vi "forecastUI.vi"(11 "ForecastDisplay in":refnum<class "ForecastDisplay.lvclass">) -> ()   [LabVIEW 2018, in "ForecastDisplay.lvclass"]
uses:
  ForecastDisplay.lvclass
panel:
  out "Waveform Chart":T1(graph)
  out "error out":errorcluster
  in  "error in (no error)":errorcluster
  # "Forecast Display"
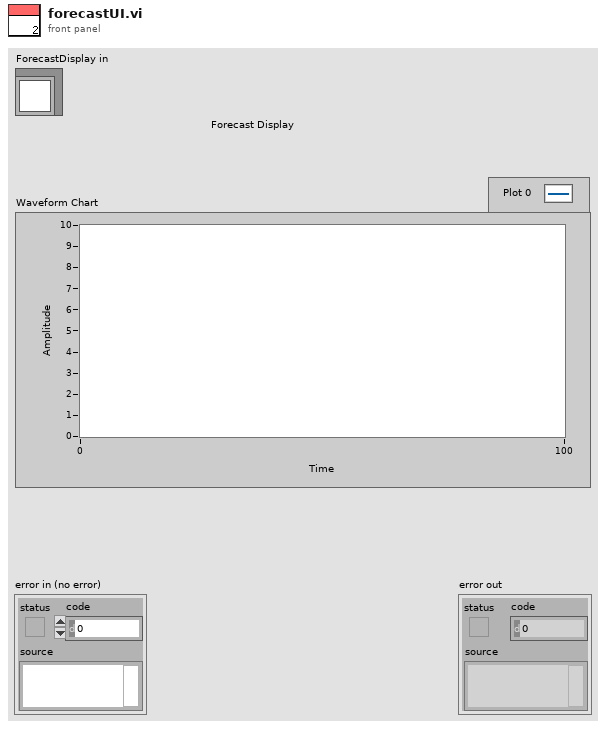
[diagram p1: front panel]
types:
  T1 = cluster{"Temperature":dbl, "Humidity":dbl, "Pressure":dbl}
  T2 = enum16{"Always On", "Always Off", "Off While Running"}
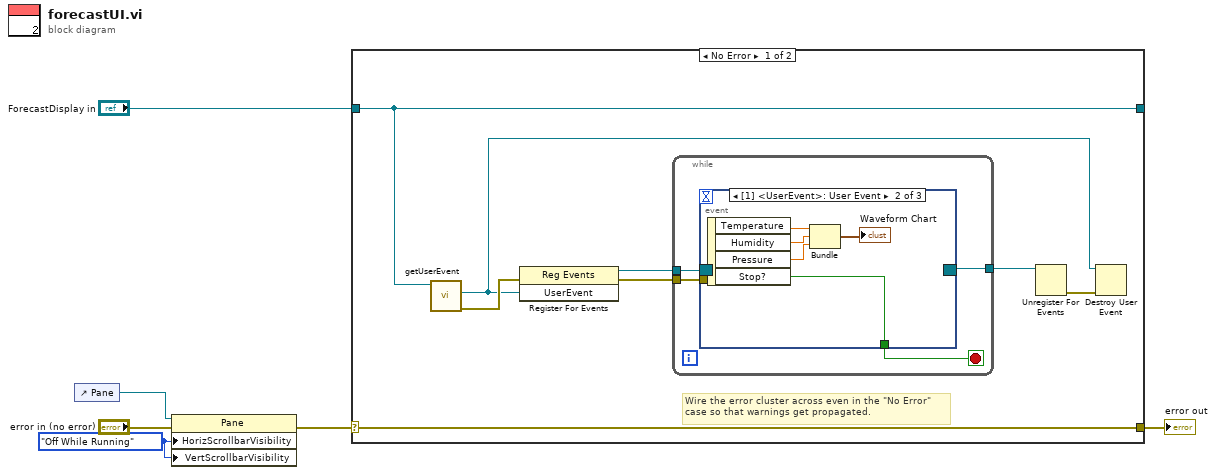
[diagram p0: block diagram]
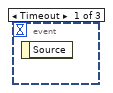
[diagram p2: hidden frame]
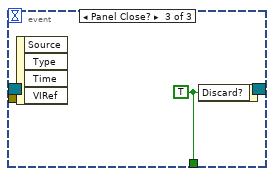
[diagram p3: hidden frame]
diagram:
  w2 = T2."Off While Running" ("Horizontal Scrollbar Visibility")
  n1 = control-ref of="Pane"() -> (w1:refnum<vi>)
  n2 = property class="Pane"(reference=w1, error in="error in (no error)", "HorizScrollbarVisibility"=w2, "VertScrollbarVisibility"=w2) -> (error out=w3:errorcluster)  [unwired: 1 out]
  n3 = case shown="No Error" w3 {
    selector: w3 -> [w14 w26]
    tunnel: [w14 w26] -> w5
    tunnel: [w10 w25] -> _
    tunnel: "ForecastDisplay in" -> [w10 w25]
    frame No Error {
      # "Wire the error cluster across even in the \"No Error\"\ncase so that warnings get propagated."
      n4 = call-dynamic "getUserEvent.vi"("ForecastDisplay in"=w10) -> ("error out"=w12:errorcluster, "UserEvent"=w8:refnum<user-event>)  [unwired: 8 in, 1 out]
      n5 = register-events(error in=w12, w8) -> (reference out=w13:refnum<event-registration>, error out=w11:errorcluster)  [unwired: 1 in]
      n6 = while {
        tunnel: w13 -> [w18]
        tunnel: w11 -> [w17]
        tunnel: [w15] -> w9
        stop <- w16 stop-if-true
        n7 = event shown="[1] <UserEvent>: User Event" {
          selector: w18 -> [_ _ _]
          dyn-events: [_ _ _] -> w15
          timeout: _ -> [_ _ _]
          tunnel: w17 -> [_ _ _]
          tunnel: [_ w19 w24] -> w16
          event Timeout {
            n8 = event-data() -> ()  [unwired: 1 in, 1 out]
          }
          event User Event {
            n9 = event-data() -> ("Temperature"=w23:dbl, "Humidity"=w22:dbl, "Pressure"=w21:dbl, "Stop?"=w19:bool)  [unwired: 1 in]
            n10 = Bundle("Temperature"=w23, "Humidity"=w22, "Pressure"=w21) -> (→"Waveform Chart":T1)  [unwired: 1 in]
          }
          event Panel Close? {
            w24 = TRUE ("Discard?")
            n11 = event-data() -> ()  [unwired: 1 in, 4 out]
            n12 = event-data("Discard?"=w24) -> ()  [unwired: 1 in, 1 out]
          }
        }
      }
      n13 = Unregister For Events(event registration refnum=w9) -> (error out=w7:errorcluster)  [unwired: 1 in]
      n14 = Destroy User Event(user event=w8, error in=w7) -> ()  [unwired: 1 out]
    }
    frame Error {
    }
  }
  "error out" <- w5
